vi "separador.vi"(2 "Entrada":u16) -> (6 "Millares":u8, 7 "Centenas":u8, 9 "Decenas":u8, 10 "Unidades":u8)   [LabVIEW 2023]
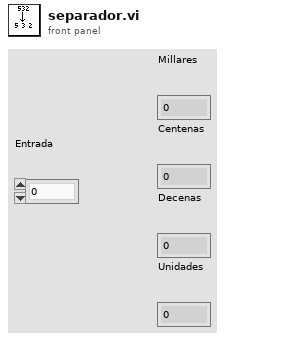
[diagram p1: front panel]
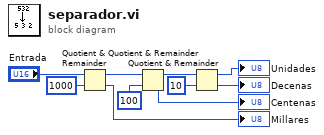
[diagram p0: block diagram]
diagram:
  n1 = Quotient & Remainder(x="Entrada", y=u16 1000) -> (x-y*floor(x/y)=w6:u16, floor(x/y)=→"Millares":u16)
  n2 = Quotient & Remainder(x=w6, y=u8 100 ("x")) -> (x-y*floor(x/y)=w3:u16, floor(x/y)=→"Centenas":u16)
  n3 = Quotient & Remainder(x=w3, y=u8 10 ("x")) -> (x-y*floor(x/y)=→"Unidades":u16, floor(x/y)=→"Decenas":u16)
